vi "Read Device Identification Response.vi"(8 "error in (no error)":errorcluster, 9 "Modbus Data Unit in":T1={"function"=1, "Data"=[]} {"function" items=["Read Discrete Inputs"=2, "Read Coils"=1, "Write Single Coil"=5, "Write Multiple Coils"=15, "Read Input Register"=4, "Read Holding Registers"=3, "Write Single Register"=6, "Write Multiple Registers"=16, "Read/Write Multiple Registers"=23, "Mask Write Register"=22, "Read FIFO Queue"=24, "Read File Record"=20, "Write File Record"=21, "Read Exception Status"=7, "Diagnostic"=8, "Get Com Event Counter"=11, "Get Com Event Log"=12, "Report Slave ID"=17, "Read Device Identification"=43]; "Data" format="%.0x"}) -> (0 "error out":errorcluster, 2 "objects":cluster{"object ID":u8, "value":string}[](array[cluster]) {"object ID" format="%x"}, 4 "next object ID":u8, 5 "conformity level":u8(ring) items=["None"=0, "Basic Stream"=1, "Regular Stream"=2, "Extended Stream"=3, "Basic Stream/Individual"=129, "Regular Stream/Individual"=130, "Extended Stream/Individual"=131], 6 "done?":bool)   [LabVIEW 2019, in "NI_modbus_upd.lvlib"]
uses:
  NI_modbus_upd.lvlib
  Ctl/MB Modbus Data Unit.ctl
  Modbus Data Unit (PDU)/Function.ctl
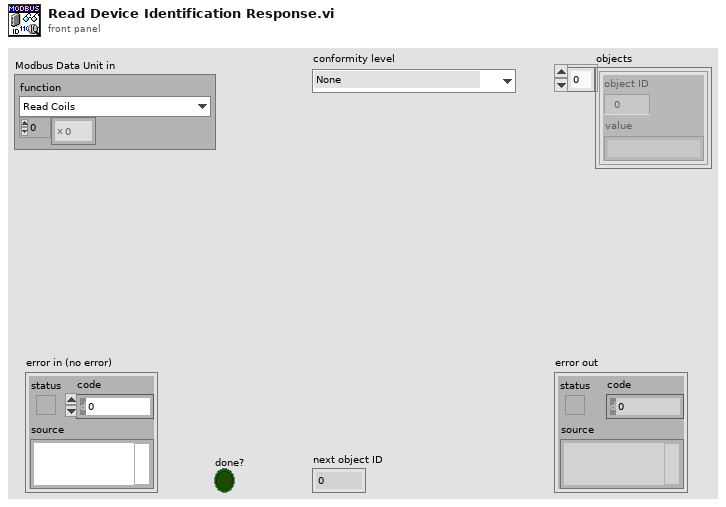
[diagram p1: front panel]
types:
  T1 = typedef "NI_modbus_upd.lvlib/MB Modbus Data Unit.ctl" = cluster{"function":T2, "Data":u8[]}
  T2 = typedef "NI_modbus_upd.lvlib/Function.ctl" = u8
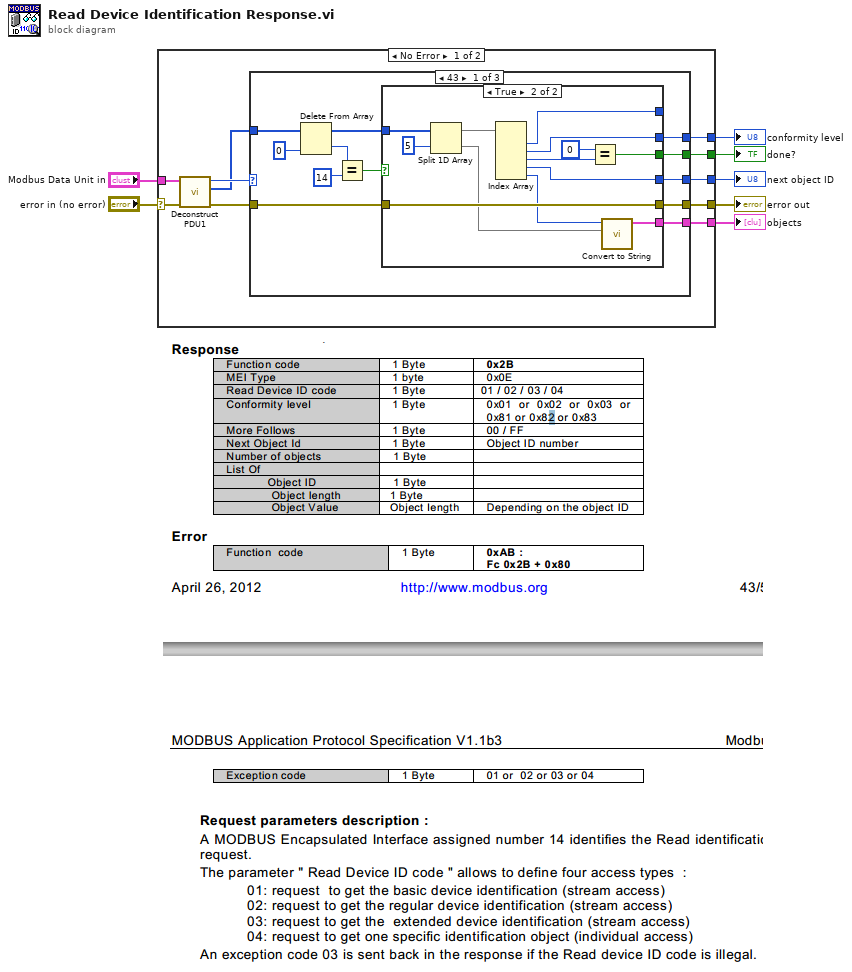
[diagram p0: block diagram]
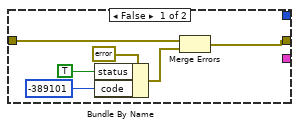
[diagram p2: hidden frame]
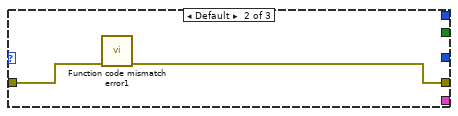
[diagram p3: hidden frame]
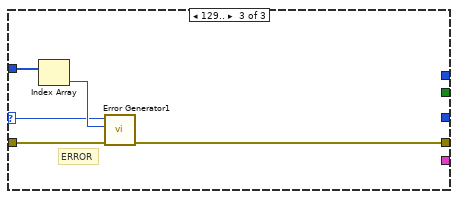
[diagram p4: hidden frame]
diagram:
  n1 = case shown="No Error" "error in (no error)" {
    selector: "error in (no error)" -> [w8 w56]
    tunnel: [w17 w56] -> w6
    tunnel: "Modbus Data Unit in" -> [w11 _]
    tunnel: [w16 _] -> w4
    tunnel: [w15 _] -> w5
    tunnel: [w14 _] -> w3
    tunnel: [w13 _] -> w2
    frame No Error {
      n2 = call "Deconstruct PDU1.vi"("error in (no error)"=w8, "Modbus Data Unit in"=w11) -> ("error out"=w9:errorcluster, "data"=w10:u8[], "function"=w12:T2)  [unwired: 7 in]
      n3 = case shown="43" w12 {
        selector: w12 -> [_ _ w51]
        tunnel: w9 -> [w27 w50 w52]
        tunnel: w10 -> [w29 _ w55]
        tunnel: [w28 w49 w54] -> w17
        tunnel: [w26 _ _] -> w16
        tunnel: [w25 _ _] -> w15
        tunnel: [w24 _ _] -> w14
        tunnel: [w23 _ _] -> w13
        frame 43 {
          n4 = Delete From Array(array=w29, index=0) -> (deleted portion=w21:u8, array with subset deleted=w22:u8[])  [unwired: 1 in]
          n5 = Equal?(x=w21, y=u8 14) -> (x = y?=w19:bool)
          n6 = case shown="True" w19 {
            tunnel: [_ w39] -> w26
            tunnel: [_ w46] -> w25
            tunnel: [_ w45] -> w24
            tunnel: [_ w44] -> w23
            tunnel: w22 -> [_ w43]
            tunnel: w27 -> [w30 w42]
            tunnel: [w31 w42] -> w28
            tunnel: [_ w36] -> _
            frame False {
              n7 = Bundle By Name(cluster=errorcluster {"status"=FALSE, "code"=0, "source"=""} ("error constant"), "status"=TRUE, "code"=-389101) -> (w34:errorcluster)
              n8 = Merge Errors(w30, w34) -> (w31:errorcluster)
            }
            frame True {
              n9 = Split 1D Array(array=w43, index=5) -> (first subarray=w47:u8[], second subarray=w38:u8[])
              n10 = Index Array(array=w47) -> (element #1=w36:u8, element #2=w46:u8, element #3=w41:u8, element #4=w45:u8, element #5=w37:u8)  [unwired: 5 in]
              n11 = Equal?(x=u8 0, y=w41) -> (x = y?=w39:bool)
              n12 = call "Convert to String.vi"("byte array"=w38, "number of objects"=w37) -> ("objects"=w44:cluster{"object ID":u8, "value":string}[])  [unwired: 9 in]
            }
          }
        }
        frame Default {
          n13 = call "Function code mismatch error1.vi"("error in (no error)"=w50) -> ("error out"=w49:errorcluster)  [unwired: 10 in]
        }
        frame 129.. {
          # "ERROR"
          n14 = Index Array(array=w55) -> (element=w53:u8)  [unwired: 1 in]
          n15 = call "Error Generator1.vi"("error in (no error)"=w52, "data return (error code)"=w53, "function return"=w51) -> ("error out"=w54:errorcluster)  [unwired: 8 in]
        }
      }
    }
    frame Error {
    }
  }
  "error out" <- w6
  "conformity level" <- w5
  "done?" <- w4
  "next object ID" <- w3
  "objects" <- w2
